vi "Init IO Ports.vi"(11 "NotifierReff":T2) -> (3 "output cluster":T1)   [LabVIEW 2013]
doc: "Initializes all I/O ports used and bundles them up for neatness.\n\nEric Schneider, April 2014"
uses:
  Data/TypeDefs/Notifiers.ctl
  Data/TypeDefs/UTM Location.ctl
  Data/TypeDefs/Sail Set Suggestions.ctl
  Data/TypeDefs/Rudder Set Suggestions.ctl
  Data/TypeDefs/OverrideInformation.ctl
  Data/TypeDefs/OverrideMode.ctl
  Data/TypeDefs/MotorSetup.ctl
  Data/TypeDefs/DynamixelSetupInfo.ctl
  Data/TypeDefs/AirmarStatus.ctl
  Data/TypeDefs/HardwareOnline.ctl
  Data/TypeDefs/DynamixelCycleTracker.ctl
  Data/TypeDefs/RC Input Values.ctl
  Classes/Waypoint/Waypoint.lvclass
  Data/TypeDefs/DamnYankeeIOPorts.ctl
  <vilib>/Instr/_visa.llb/VISA Configure Serial Port (Instr).vi
  <instrlib>/Dynamixel Motor/Dynamixel Motor.lvlib
  <vilib>/rvi/interface/nirviOpenFPGA/nirviOpenFPGA.xnode
  FPGA_Code/DamnYankeeFPGA.vi
panel:
  out "Motors IDs Found":u8[](array[numeric])
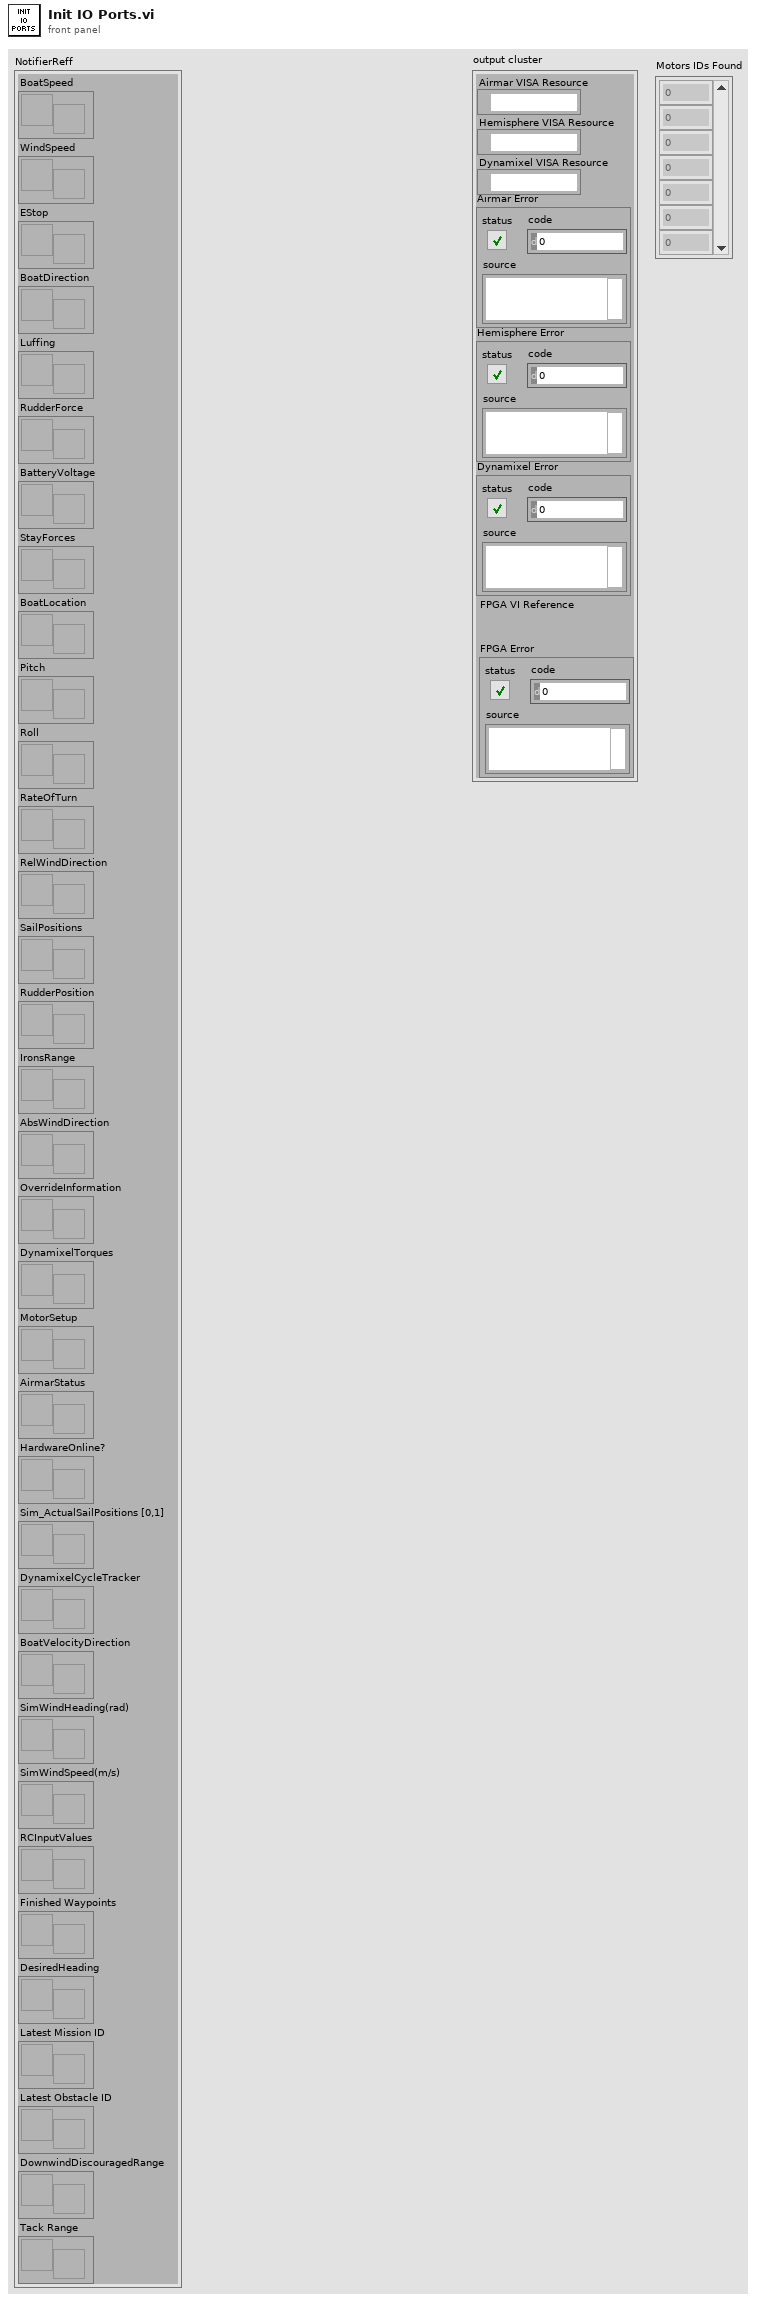
[diagram p1: front panel]
types:
  T1 = typedef "DamnYankeeIOPorts.ctl" = cluster{"Airmar VISA Resource":refnum<visa-resource-name>, "Hemisphere VISA Resource":refnum<visa-resource-name>, "Dynamixel VISA Resource":refnum<visa-resource-name>, "Airmar Error":errorcluster, "Hemisphere Error":errorcluster, "Dynamixel Error":errorcluster, "FPGA VI Reference":refnum<k20>, "FPGA Error":errorcluster}
  T2 = typedef "Notifiers.ctl" = cluster{"BoatSpeed":refnum<notifier>, "WindSpeed":refnum<notifier>, "EStop":refnum<notifier>, "BoatDirection":refnum<notifier>, "Luffing":refnum<notifier>, "RudderForce":refnum<notifier>, "BatteryVoltage":refnum<notifier>, "StayForces":refnum<notifier>, "BoatLocation":refnum<notifier>, "Pitch":refnum<notifier>, "Roll":refnum<notifier>, "RateOfTurn":refnum<notifier>, "RelWindDirection":refnum<notifier>, "SailPositions":refnum<notifier>, "RudderPosition":refnum<notifier>, "IronsRange":refnum<notifier>, "AbsWindDirection":refnum<notifier>, "OverrideInformation":refnum<notifier>, "DynamixelTorques":refnum<notifier>, "MotorSetup":refnum<notifier>, "AirmarStatus":refnum<notifier>, "HardwareOnline?":refnum<notifier>, "Sim_ActualSailPositions [0,1]":refnum<notifier>, "DynamixelCycleTracker":refnum<notifier>, "BoatVelocityDirection":refnum<notifier>, "SimWindHeading(rad)":refnum<notifier>, "SimWindSpeed(m/s)":refnum<notifier>, "RCInputValues":refnum<notifier>, "Finished Waypoints":refnum<notifier>, "DesiredHeading":refnum<notifier>, "Latest Mission ID":refnum<notifier>, "Latest Obstacle ID":refnum<notifier>, "DownwindDiscouragedRange":refnum<notifier>, "Tack Range":refnum<notifier>}
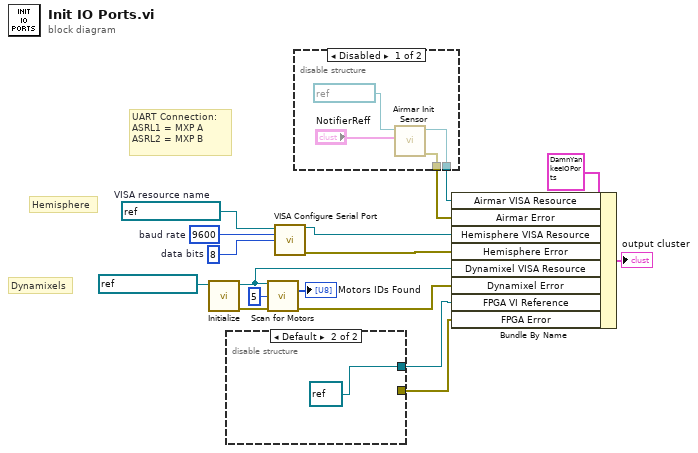
[diagram p0: block diagram]
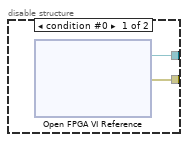
[diagram p3: hidden frame]
diagram:
  w3 = u16 8  # data bits
  w4 = u32 9600  # baud rate
  w2 = refnum<visa-resource-name> "ASRL1::INSTR"  # VISA resource name
  # "Dynamixels"
  # "Hemisphere"
  # "UART Connection:\nASRL1 = MXP A \nASRL2 = MXP B"
  n1 = call <instrlib>:"Initialize.vi"("VISA resource name"=refnum<visa-resource-name> "ASRL3::INSTR") -> ("error out"=w8:errorcluster, "VISA resource name out"=w10:refnum<visa-resource-name>)  [unwired: 9 in]
  n2 = disable-structure shown="Default" {
    disable-tunnel: [w19 refnum<k20> refnum ("FPGA VI Reference")] -> w1
    disable-tunnel: [w18 _] -> w5
    frame condition #0 {
      n3 = xnode "Open FPGA VI Reference"() -> ("FPGA VI Reference Out"=w19:refnum<k20>, "error out"=w18:errorcluster)  [unwired: 2 in]
    }
    frame condition #1 (active) {
    }
  }
  n4 = call <instrlib>:"Scan for Motors.vi"("VISA resource name"=w10, "Ending ID (253)"=u8 5, "error in (no error)"=w8) -> ("Motors IDs Found"=→"Motors IDs Found":u8[], "error out"=w7:errorcluster)  [unwired: 10 in, 1 out]
  n5 = call-poly "VISA Configure Serial Port"("VISA resource name"=w2, "baud rate (9600)"=w4, "data bits (8)"=w3) -> ("VISA resource name out"=w16:refnum<visa-resource-name>, "error out"=w15:errorcluster)  [unwired: 11 in]
  n6 = disable-structure shown="Disabled" {
    disable-tunnel: [w24 _] -> w14
    disable-tunnel: [w23 _] -> w13
    frame Disabled {
      n7 = call "Airmar Init Sensor.vi"("NotifierReff"="NotifierReff", "VISA Refnum in"=refnum<visa-resource-name> "COM1") -> ("error out"=w23:errorcluster, "VISA Refnum out"=w24:refnum<visa-resource-name>)  [unwired: 7 in, 1 out]
    }
    frame Enabled {
    }
  }
  n8 = Bundle By Name(cluster=T1 {"Airmar VISA Resource"="", "Hemisphere VISA Resource"="", "Dynamixel VISA Resource"="", "Airmar Error"={"status"=FALSE, "code"=0, "source"=""}, "Hemisphere Error"={"status"=FALSE, "code"=0, "source"=""}, "Dynamixel Error"={"status"=FALSE, "code"=0, "source"=""}, "FPGA VI Reference"=refnum, "FPGA Error"={"status"=FALSE, "code"=0, "source"=""}}, "Airmar VISA Resource"=w14, "Airmar Error"=w13, "Hemisphere VISA Resource"=w16, "Hemisphere Error"=w15, "Dynamixel VISA Resource"=w10, "Dynamixel Error"=w7, "FPGA VI Reference"=w1, "FPGA Error"=w5) -> (→"output cluster":T1)
